vi "LaunchRoot.vi"   [LabVIEW 2020]
uses:
  <vilib>/ActorFramework/Actor/Actor.lvclass
  TopUI/TopUI/TopUI.lvclass
panel:
  # "Launch TopUI"
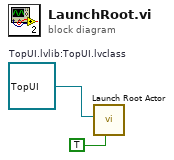
[diagram p0: block diagram]
diagram:
  w1 = refnum<class "TopUI.lvclass"> refnum  # TopUI.lvlib:TopUI.lvclass
  n1 = call <vilib>:"Launch Root Actor.vi"("Open Actor Core front panel? (F)"=TRUE, "Actor"=w1) -> ()  [unwired: 8 in, 2 out]
